vi "Senior Project.vi"() -> ()   [LabVIEW 2010]
panel:
  in  "Scan Enum":enum16{""}(ring)
  in  "Manual Scan >>":bool
  in  "Manual Scan >":bool
  in  "< Manual Scan":bool
  in  "<< Manual Scan":bool
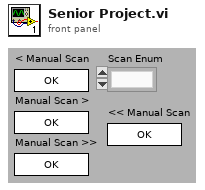
[diagram p1: front panel]
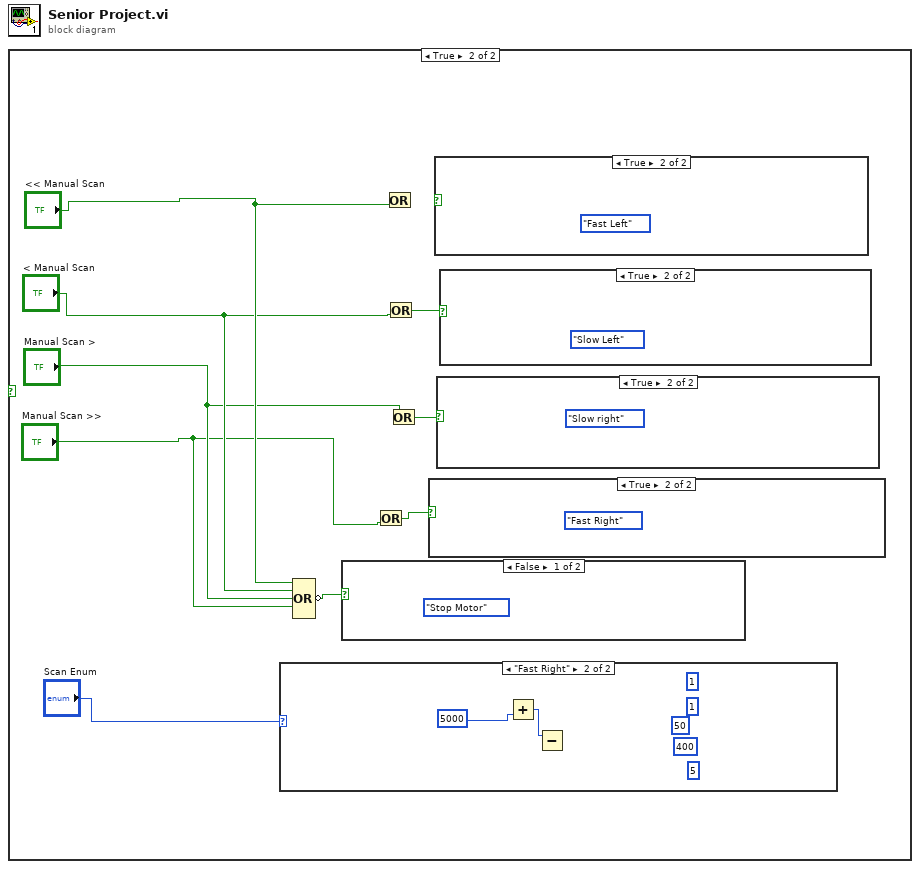
[diagram p0: block diagram]
diagram:
  n1 = case shown="True" {
    selector: _ -> [_ _]
    frame False {
    }
    frame True {
      n2 = case shown="\"Fast Right\"" "Scan Enum" {
        frame "", Default {
        }
        frame 1 {
          (unwired) 50
          (unwired) 1
          (unwired) 1
          (unwired) 400
          (unwired) 5
          n3 = Add(y=5000) -> (x+y=w11:i32)  [unwired: 1 in]
          n4 = Subtract(x=w11) -> ()  [unwired: 1 in, 1 out]
        }
      }
      n5 = Compound Arithmetic op=OR("<< Manual Scan", "< Manual Scan", "Manual Scan >", "Manual Scan >>") -> (invert w6:bool)  [unwired: 1 in]
      n6 = case shown="False" w6 {
        frame False {
          (unwired) enum16{"Stop Motor", ""}."Stop Motor" ("Enum")
        }
        frame True {
        }
      }
      n7 = Or(y="Manual Scan >>") -> (x .or. y?=w7:bool)  [unwired: 1 in]
      n8 = Or(y="<< Manual Scan") -> ()  [unwired: 1 in, 1 out]
      n9 = Or(y="< Manual Scan") -> (x .or. y?=w9:bool)  [unwired: 1 in]
      n10 = Or(y="Manual Scan >") -> (x .or. y?=w8:bool)  [unwired: 1 in]
      n11 = case shown="True" w7 {
        frame False {
        }
        frame True {
          (unwired) enum16{"Fast Right", ""}."Fast Right" ("Enum")
        }
      }
      n12 = case shown="True" {
        selector: _ -> [_ _]
        frame False {
        }
        frame True {
          (unwired) enum16{"Fast Left", ""}."Fast Left" ("Enum")
        }
      }
      n13 = case shown="True" w8 {
        frame False {
        }
        frame True {
          (unwired) enum16{"Slow right", ""}."Slow right" ("Enum")
        }
      }
      n14 = case shown="True" w9 {
        frame False {
        }
        frame True {
          (unwired) enum16{"Slow Left", ""}."Slow Left" ("Enum")
        }
      }
    }
  }
